vi "Robotics Environment Simulator.vi"() -> ()   [LabVIEW 2018]
doc: "This VI starts and stops the environment simulator and serves as the master VI for your simulation code. Open and run this VI to display the environment simulator, or open the block diagram to view or modify simulation code."
uses:
  <vilib>/robotics/Controls/Simulator Display/Simulator Display.xctl
  <vilib>/robotics/Simulator/Engine/ctl/Step Mode.ctl
  <vilib>/Platform/TimedLoop/XDataNode/timing_clust.ctl
  <vilib>/Platform/TimedLoop/XDataNode/nitl_modes.ctl
  <vilib>/Platform/TimedLoop/XDataNode/wakeup.ctl
  <vilib>/Platform/TimedLoop/XDataNode/XDataNode.xnode
  <instrlib>/DC Motor Controller/HAIOL/DC Motor Controller.lvclass
  <vilib>/robotics/Simulator/NI_Robotics_Simulator.lvlib
  <vilib>/Platform/TimedLoop/XDataNode/XDNodeRunTimeDep.lvlib
  <instrlib>/DC Motor Controller/HAIOL/Simulator/DC Motor Controller Simulator.lvclass
panel:
  in  "Simulator Display":refnum<vi>(xcontrol)
  in  "manifest filename":string="Robotics Environment Simulator.xml"
  in  "stop":bool
  # "* Press the Run button to display the Robotics Environment Simulator.\n* Select Window>>Show Block Diagram or press <Ctrl-E> to view the block diagram, where you can add or modify simulation code. Add controls and indicators to the front panel of this VI to pass data into and out of the simulation code.\n* The manifest file must exist in same directory as the .lvproj file."
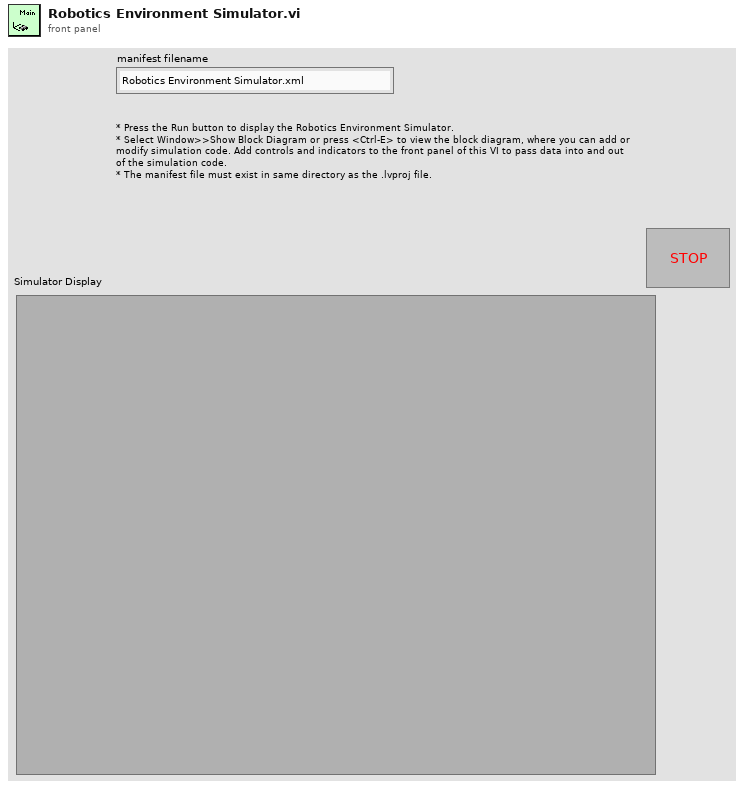
[diagram p1: front panel]
types:
  T1 = cluster{"Robot ID":string, "Device Label":string}
  T2 = typedef "NI_Robotics_Simulator.lvlib/Step Mode.ctl" = u16
  T3 = typedef "XDNodeRunTimeDep.lvlib/timing_clust.ctl" = cluster{"Expected End [f-1]":u64, "Actual End [f-1]":u64, "Finished Late? [f-1]":bool, "Expected End [i-1]":u64, "Actual End [i-1]":u64, "Finished Late? [i-1]":bool, "Expected Start [i]":u64, "Actual Start [i]":u64, "Expected Start [f]":u64, "Actual Start [f]":u64, "Source Name":string, "Structure Name":string, "Period":i64, "Deadline":i64, "Offset":i64, "Start":i64, "Priority":i32, "Timeout":i32, "Mode":T4, "Wakeup Reason":T5, "Error":errorcluster, "Source Type":string, "Secondary Source Type":string, "Global End Time":u64, "Global Start Time":u64, "Frame Duration":u64, "Iteration Duration":u64, "Assigned CPU":i32, "I/O Scan Engine Mode":u32}
  T4 = typedef "XDNodeRunTimeDep.lvlib/nitl_modes.ctl" = enum32{"No Change", "Process missed periods, maintain original phase", "Discard missed periods, maintain original phase", "Process missed periods, ignore original phase", "Discard missed periods, ignore original phase"}
  T5 = typedef "XDNodeRunTimeDep.lvlib/wakeup.ctl" = enum32{"Normal", "Aborted", "Asynchronous wakeup", "Timing source error", "Timed loop error", "Timeout"}
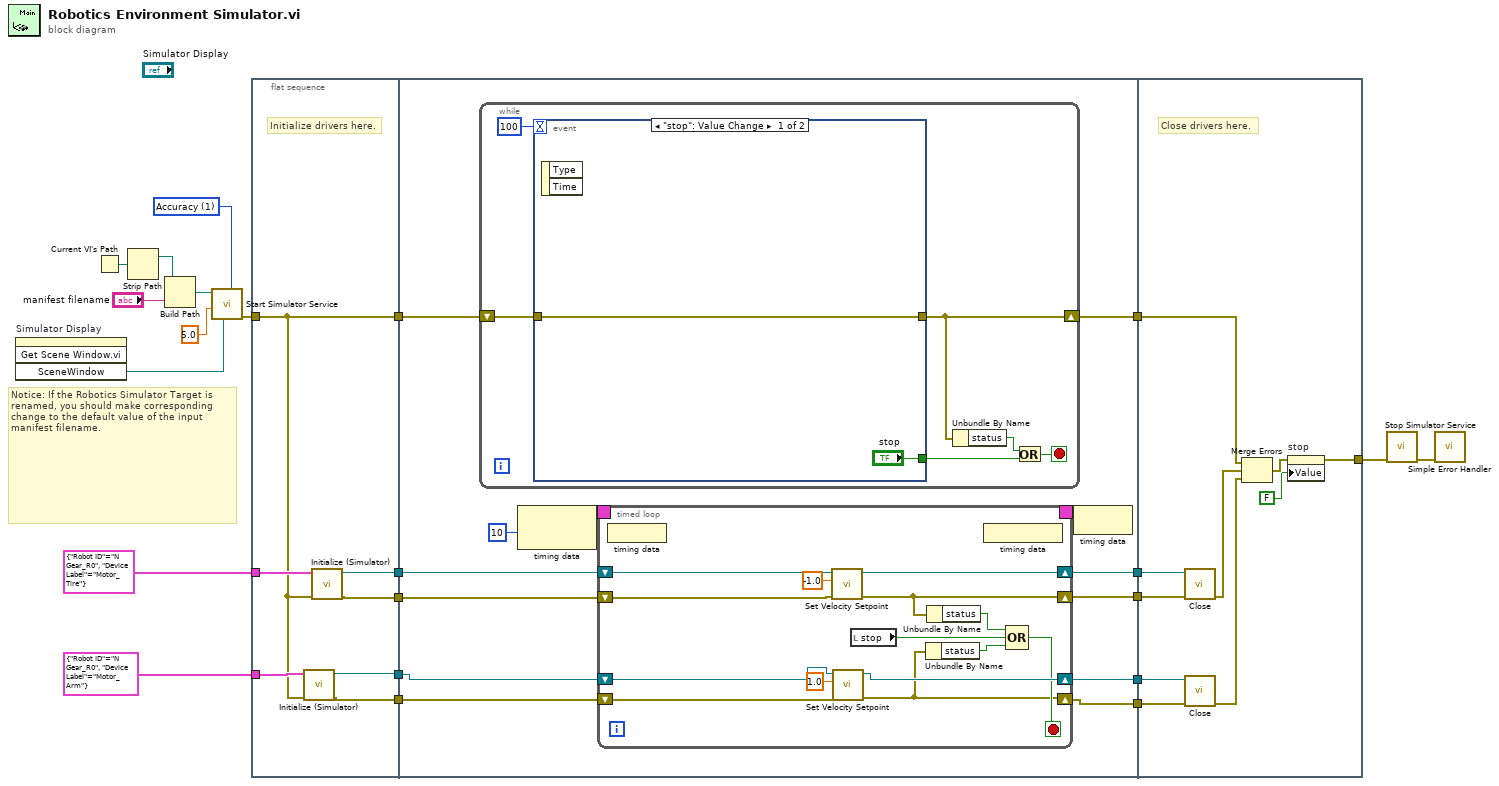
[diagram p0: block diagram]
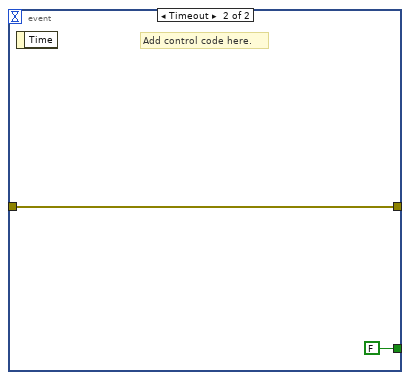
[diagram p2: hidden frame]
diagram:
  w12 = T2 1 items=["Performance", "Accuracy"] ("step mode")
  # "Notice: If the Robotics Simulator Target is renamed, you should make corresponding change to the default value of the input manifest filename."
  n1 = invoke on="Simulator Display" class="Simulator Display (strict)" method="Get Scene Window.vi"() -> ("SceneWindow"=w13:refnum<vi>)  [unwired: 4 in, 3 out]
  n2 = Current VI's Path() -> (path=w21:path)
  n3 = Strip Path(path=w21) -> (stripped path=w20:path)  [unwired: 1 out]
  n4 = Build Path(base path=w20, name or relative path="manifest filename") -> (appended path=w19:path)
  n5 = call <vilib>:"Start Simulator Service.vi"("step mode"=w12, "3D picture refnum"=w13, "step size (ms)"=5.0 ("stepsize(ms)"), "manifest file"=w19) -> ("error out"=w16:errorcluster)  [unwired: 7 in]
  n6 = flat-sequence {
    tunnel: w16 -> [w23]
    tunnel: [w23] -> w15
    tunnel: T1 {"Robot ID"="N Gear_R0", "Device Label"="Motor_Tire"} ("Device ID") -> [w29]
    tunnel: T1 {"Robot ID"="N Gear_R0", "Device Label"="Motor_Arm"} ("Device ID") -> [w26]
    tunnel: [w28] -> w9
    tunnel: [w27] -> w8
    tunnel: [w24] -> w7
    tunnel: [w25] -> w6
    tunnel: w15 -> [w41]
    tunnel: [w42] -> w14
    tunnel: w9 -> [w37]
    tunnel: w8 -> [w32]
    tunnel: w7 -> [w36]
    tunnel: w6 -> [w35]
    tunnel: [w34] -> w5
    tunnel: [w33] -> w4
    tunnel: [w30] -> w3
    tunnel: [w31] -> w2
    tunnel: w14 -> [w73]
    tunnel: w5 -> [w82]
    tunnel: w4 -> [w81]
    tunnel: w3 -> [w80]
    tunnel: w2 -> [w79]
    tunnel: [w74] -> w1
    frame #0 {
      # "Initialize drivers here."
      n7 = call <instrlib>:"Initialize (Simulator).vi"("error in (no error)"=w23, "Device ID"=w26) -> ("error out"=w25:errorcluster, "DC Motor Controller out"=w24:refnum<class "DC Motor Controller.lvclass">)  [unwired: 8 in]
      n8 = call <instrlib>:"Initialize (Simulator).vi"("error in (no error)"=w23, "Device ID"=w29) -> ("error out"=w27:errorcluster, "DC Motor Controller out"=w28:refnum<class "DC Motor Controller.lvclass">)  [unwired: 8 in]
    }
    frame #1 {
      n9 = while {
        shift-right: [w64] -> w42
        shift-left: w41 -> [w67]
        stop <- w65 stop-if-true
        n10 = event shown="[0] \"stop\": Value Change" {
          selector: _ -> [_ _]
          dyn-events: _ -> [_ _]
          timeout: 100 -> [_ _]
          tunnel: ["stop" FALSE ("stop")] -> w66
          tunnel: [w69 w72] -> w64
          tunnel: w67 -> [w69 w72]
          event "stop": Value Change {
            n11 = event-data() -> ()  [unwired: 1 in, 2 out]
          }
          event Timeout {
            # "Add control code here."
            n12 = event-data() -> ()  [unwired: 1 in, 1 out]
          }
        }
        n13 = Unbundle By Name(w64) -> ("status"=w63:bool)
        n14 = Or(x=w63, y=w66) -> (x .or. y?=w65:bool)
      }
      n15 = node-c288(i64 10 ("Period")) -> (w40:T3)
      n16 = timed-loop {
        timing: w40 -> [_]
        timing-out: [_] -> w39
        shift-right: [w53] -> w34
        shift-left: w37 -> [w56]
        shift-right: [w48] -> w31
        shift-left: w32 -> [w51]
        shift-right: [w52] -> w33
        shift-left: w36 -> [w55]
        shift-right: [w43] -> w30
        shift-left: w35 -> [w54]
        stop <- w44 stop-if-true
        n17 = node-c288() -> ()  [unwired: 1 in]
        n18 = call-dynamic "Set Velocity Setpoint.vi"("error in (no error)"=w51, "CCW Velocity (0 rad/s)"=-1.0, "DC Motor Controller in"=w56) -> ("error out"=w48:errorcluster, "DC Motor Controller out"=w53:refnum<class "DC Motor Controller.lvclass">)  [unwired: 7 in]
        n19 = call-dynamic "Set Velocity Setpoint.vi"("error in (no error)"=w54, "CCW Velocity (0 rad/s)"=1.0, "DC Motor Controller in"=w55) -> ("error out"=w43:errorcluster, "DC Motor Controller out"=w52:refnum<class "DC Motor Controller.lvclass">)  [unwired: 7 in]
        n20 = local read "stop"() -> (w45:bool)
        n21 = Unbundle By Name(w43) -> ("status"=w47:bool)
        n22 = Unbundle By Name(w48) -> ("status"=w46:bool)
        n23 = node-c288() -> ()  [unwired: 1 out]
        n24 = Compound Arithmetic op=OR(w46, w45, w47) -> (w44:bool)
      }
      n25 = node-c288(w39) -> ()
    }
    frame #2 {
      # "Close drivers here."
      n26 = call-dynamic "Close.vi"("error in (no error)"=w79, "DC Motor Controller in"=w82) -> ("error out"=w78:errorcluster)  [unwired: 9 in]
      n27 = call-dynamic "Close.vi"("error in (no error)"=w80, "DC Motor Controller in"=w81) -> ("error out"=w77:errorcluster)  [unwired: 9 in]
      n28 = Merge Errors(w73, w78, w77) -> (w76:errorcluster)
      n29 = property on="stop" class="Bool (strict)"(error in=w76, "Value"=FALSE ("stop")) -> (error out=w74:errorcluster)  [unwired: 1 in, 1 out]
    }
  }
  n30 = call <vilib>:"Stop Simulator Service.vi"("error in (no error)"=w1) -> ("error out"=w17:errorcluster)  [unwired: 10 in]
  n31 = call <vilib>:"Simple Error Handler.vi"("error in (no error)"=w17) -> ()  [unwired: 4 in, 5 out]
